vi "VSG-AMPL_REF_STATE.vi"(6 "Ref State ON(T)":bool=TRUE, 8 "error in":errorcluster {"code" format="%.0x"}, 11 "Session In":refnum<visa-resource-name>="GPIB0::18::INSTR") -> (0 "error out":errorcluster {"code" format="%.0x"}, 3 "Session Out":refnum<visa-resource-name>)   [LabVIEW 2018]
doc: "Set/Get the ESG RF Amplitude in current units."
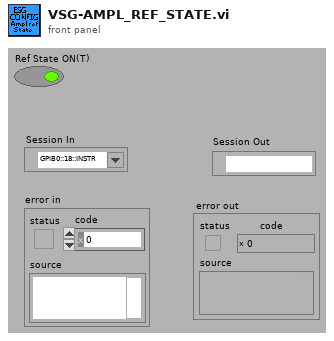
[diagram p1: front panel]
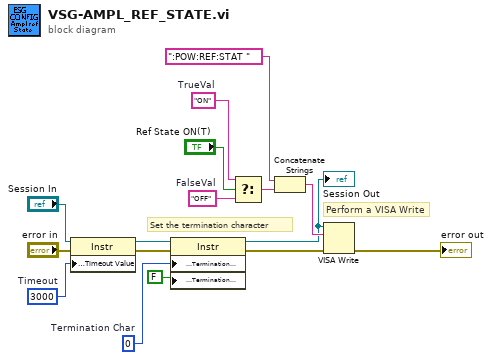
[diagram p0: block diagram]
diagram:
  w8 = u8 0  # Termination Char
  w12 = u32 3000  # Timeout
  w13 = "OFF"  # FalseVal
  w14 = "ON"  # TrueVal
  # "Perform a VISA Write"
  # "Set the termination character"
  n1 = property class="Instr"(reference="Session In", error in="error in", "General Settings:Timeout Value"=w12) -> (reference out=w7:refnum<visa-resource-name>, error out=w10:errorcluster)
  n2 = property class="Instr"(reference=w7, error in=w10, "Message Based Settings:Termination Character"=w8, "Message Based Settings:Termination Character Enable"=FALSE ("enable")) -> (reference out=w1:refnum<visa-resource-name>, error out=w9:errorcluster)
  "Session Out" <- w1
  n3 = Select(t=w14, s="Ref State ON(T)", f=w13) -> (s? t:f=w5:string)
  n4 = Concatenate Strings(":POW:REF:STAT " ("staticText"), w5) -> (w2:string)
  n5 = VISA Write(VISA resource name=w1, write buffer=w2, error in (no error)=w9) -> (error out=→"error out":errorcluster)  [unwired: 2 out]
